vi "channel-analyzer.vi"() -> ()   [LabVIEW 2023]
uses:
  <vilib>/Utility/NIReport.llb/Report Type.ctl
  <vilib>/Platform/TimedLoop/XDataNode/timing_clust.ctl
  <vilib>/Platform/TimedLoop/XDataNode/nitl_modes.ctl
  <vilib>/Platform/TimedLoop/XDataNode/wakeup.ctl
  e44e8500-82ed-4d51-b0d7-703651abc422.vi
  <vilib>/Utility/NIReport.llb/Append Numeric Table to Report (wrap).vi
  <vilib>/Instr/_visa.llb/VISA Configure Serial Port (Instr).vi
  <vilib>/express/express analysis/Spectral/Block/exnSpectralBlock spectral measurements peak poly.vi
  <vilib>/express/express analysis/Spectral/Block/exnSpectralBlock spectral measurements peak WFM.vi
  <vilib>/platform/TimedLoop/XDataNode/XDataNode.xnode
  <vilib>/express/express analysis/Spectral/XNode/ExpressSpectralMeasurementsBlockNode.xnode
  <vilib>/Utility/NIReport.llb/NI_report.lvclass
  <vilib>/Utility/NIReport.llb/Excel/NI_Excel.lvclass
  <vilib>/Utility/NIReport.llb/NI_ReportGenerationCore.lvlib
  <vilib>/Platform/TimedLoop/XDataNode/XDNodeRunTimeDep.lvlib
panel:
  in  "Magnitude (V)":sgl min=0 max=3.3
  out "Block Size Indicator":u32
  in  "Block Size":u16(knob) min=6 max=12 scale=6.0..12.0
  in  "Start":bool
  in  "Stop Frequency (Hz)":sgl min=0 max=25000
  in  "Frequency Step (Hz)":sgl min=6.103516 max=24000
  in  "Save":bool
  in  "Start Frequency (Hz)":sgl min=1 max=25000
  out "Frequency Domain Indicator":cluster{"f0":dbl, "df":dbl, "magnitude":dbl[]}
  out "Time Domain Indicator":waveform(dbl)
  in  "Resolution (Bits)":u8 min=5 max=9
  in  "Connect":bool
  in  "Stop":bool
  in  "Reference Voltage (V)":sgl min=0
  in  "Baud Rate (BPS)":u32
  in  "COM Port":refnum<visa-resource-name>
  in  "Sampling Rate (Hz)":sgl min=0
  in  "Tab Control":enum32{"Oscilloscope", "Analyzer"}(tab)
  out "Time Domain":waveform(dbl)(graph)
  out "Frequency Domain":waveform(dbl)[](graph)
  out "Bode Plot":waveform(dbl)[](graph)
  # "CHANNEL ANALYZER"
  # "SETTINGS"
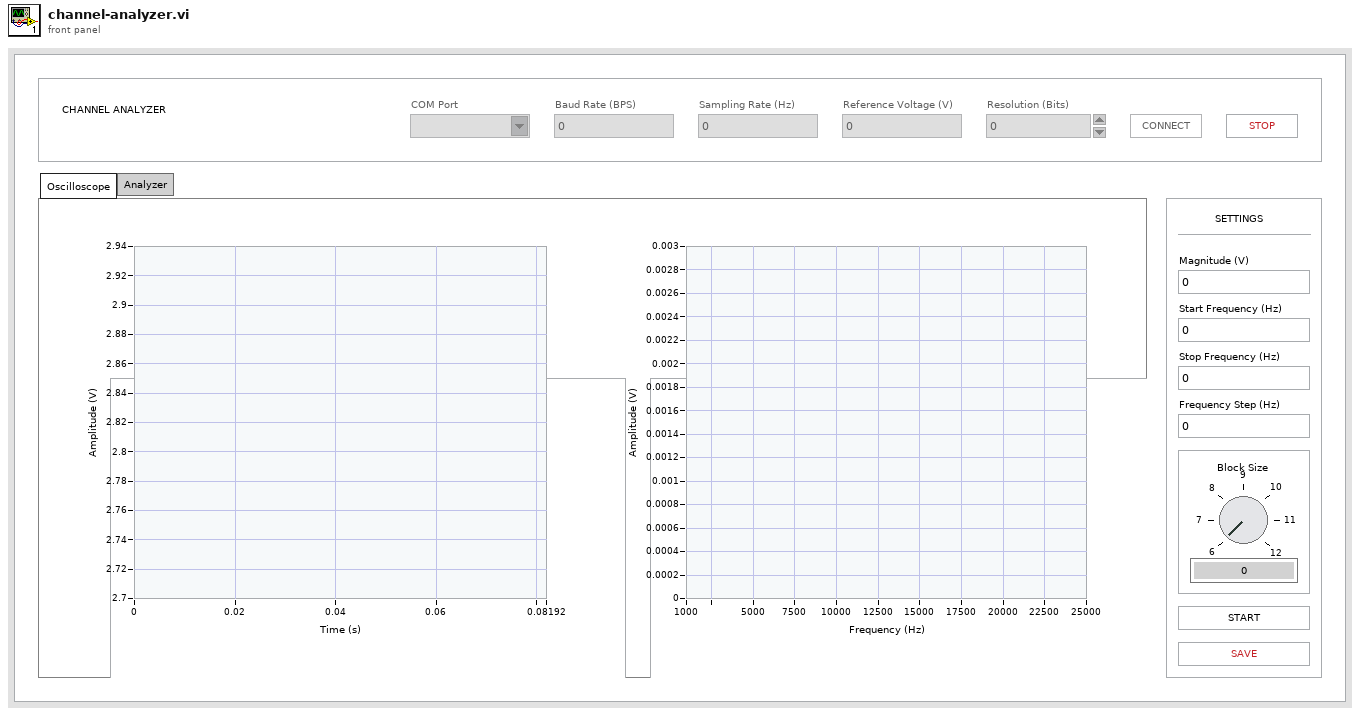
[diagram p1: front panel]
types:
  T1 = cluster{"averaging mode":u16, "weighting mode":u16, "number of averages":u32}
  T2 = cluster{"dB On (F)":bool, "unwrap phase (F)":bool, "convert to degree (F)":bool}
  T3 = enum8{"Enabled", "Disabled", "Disabled and Grayed Out"}
  T4 = typedef "NI_ReportGenerationCore.lvlib/Report Type.ctl" = enum16{"HTML", "Word", "Excel"}
  T5 = typedef "XDNodeRunTimeDep.lvlib/timing_clust.ctl" = cluster{"Expected End [f-1]":u64, "Actual End [f-1]":u64, "Finished Late? [f-1]":bool, "Expected End [i-1]":u64, "Actual End [i-1]":u64, "Finished Late? [i-1]":bool, "Expected Start [i]":u64, "Actual Start [i]":u64, "Expected Start [f]":u64, "Actual Start [f]":u64, "Source Name":string, "Structure Name":string, "Period":i64, "Deadline":i64, "Offset":i64, "Start":i64, "Priority":i32, "Timeout":i32, "Mode":T6, "Wakeup Reason":T7, "Error":errorcluster, "Source Type":string, "Secondary Source Type":string, "Global End Time":u64, "Global Start Time":u64, "Frame Duration":u64, "Iteration Duration":u64, "Assigned CPU":i32, "I/O Scan Engine Mode":u32}
  T6 = typedef "XDNodeRunTimeDep.lvlib/nitl_modes.ctl" = enum32{"No Change", "Process missed periods, maintain original phase", "Discard missed periods, maintain original phase", "Process missed periods, ignore original phase", "Discard missed periods, ignore original phase"}
  T7 = typedef "XDNodeRunTimeDep.lvlib/wakeup.ctl" = enum32{"Normal", "Aborted", "Asynchronous wakeup", "Timing source error", "Timed loop error", "Timeout"}
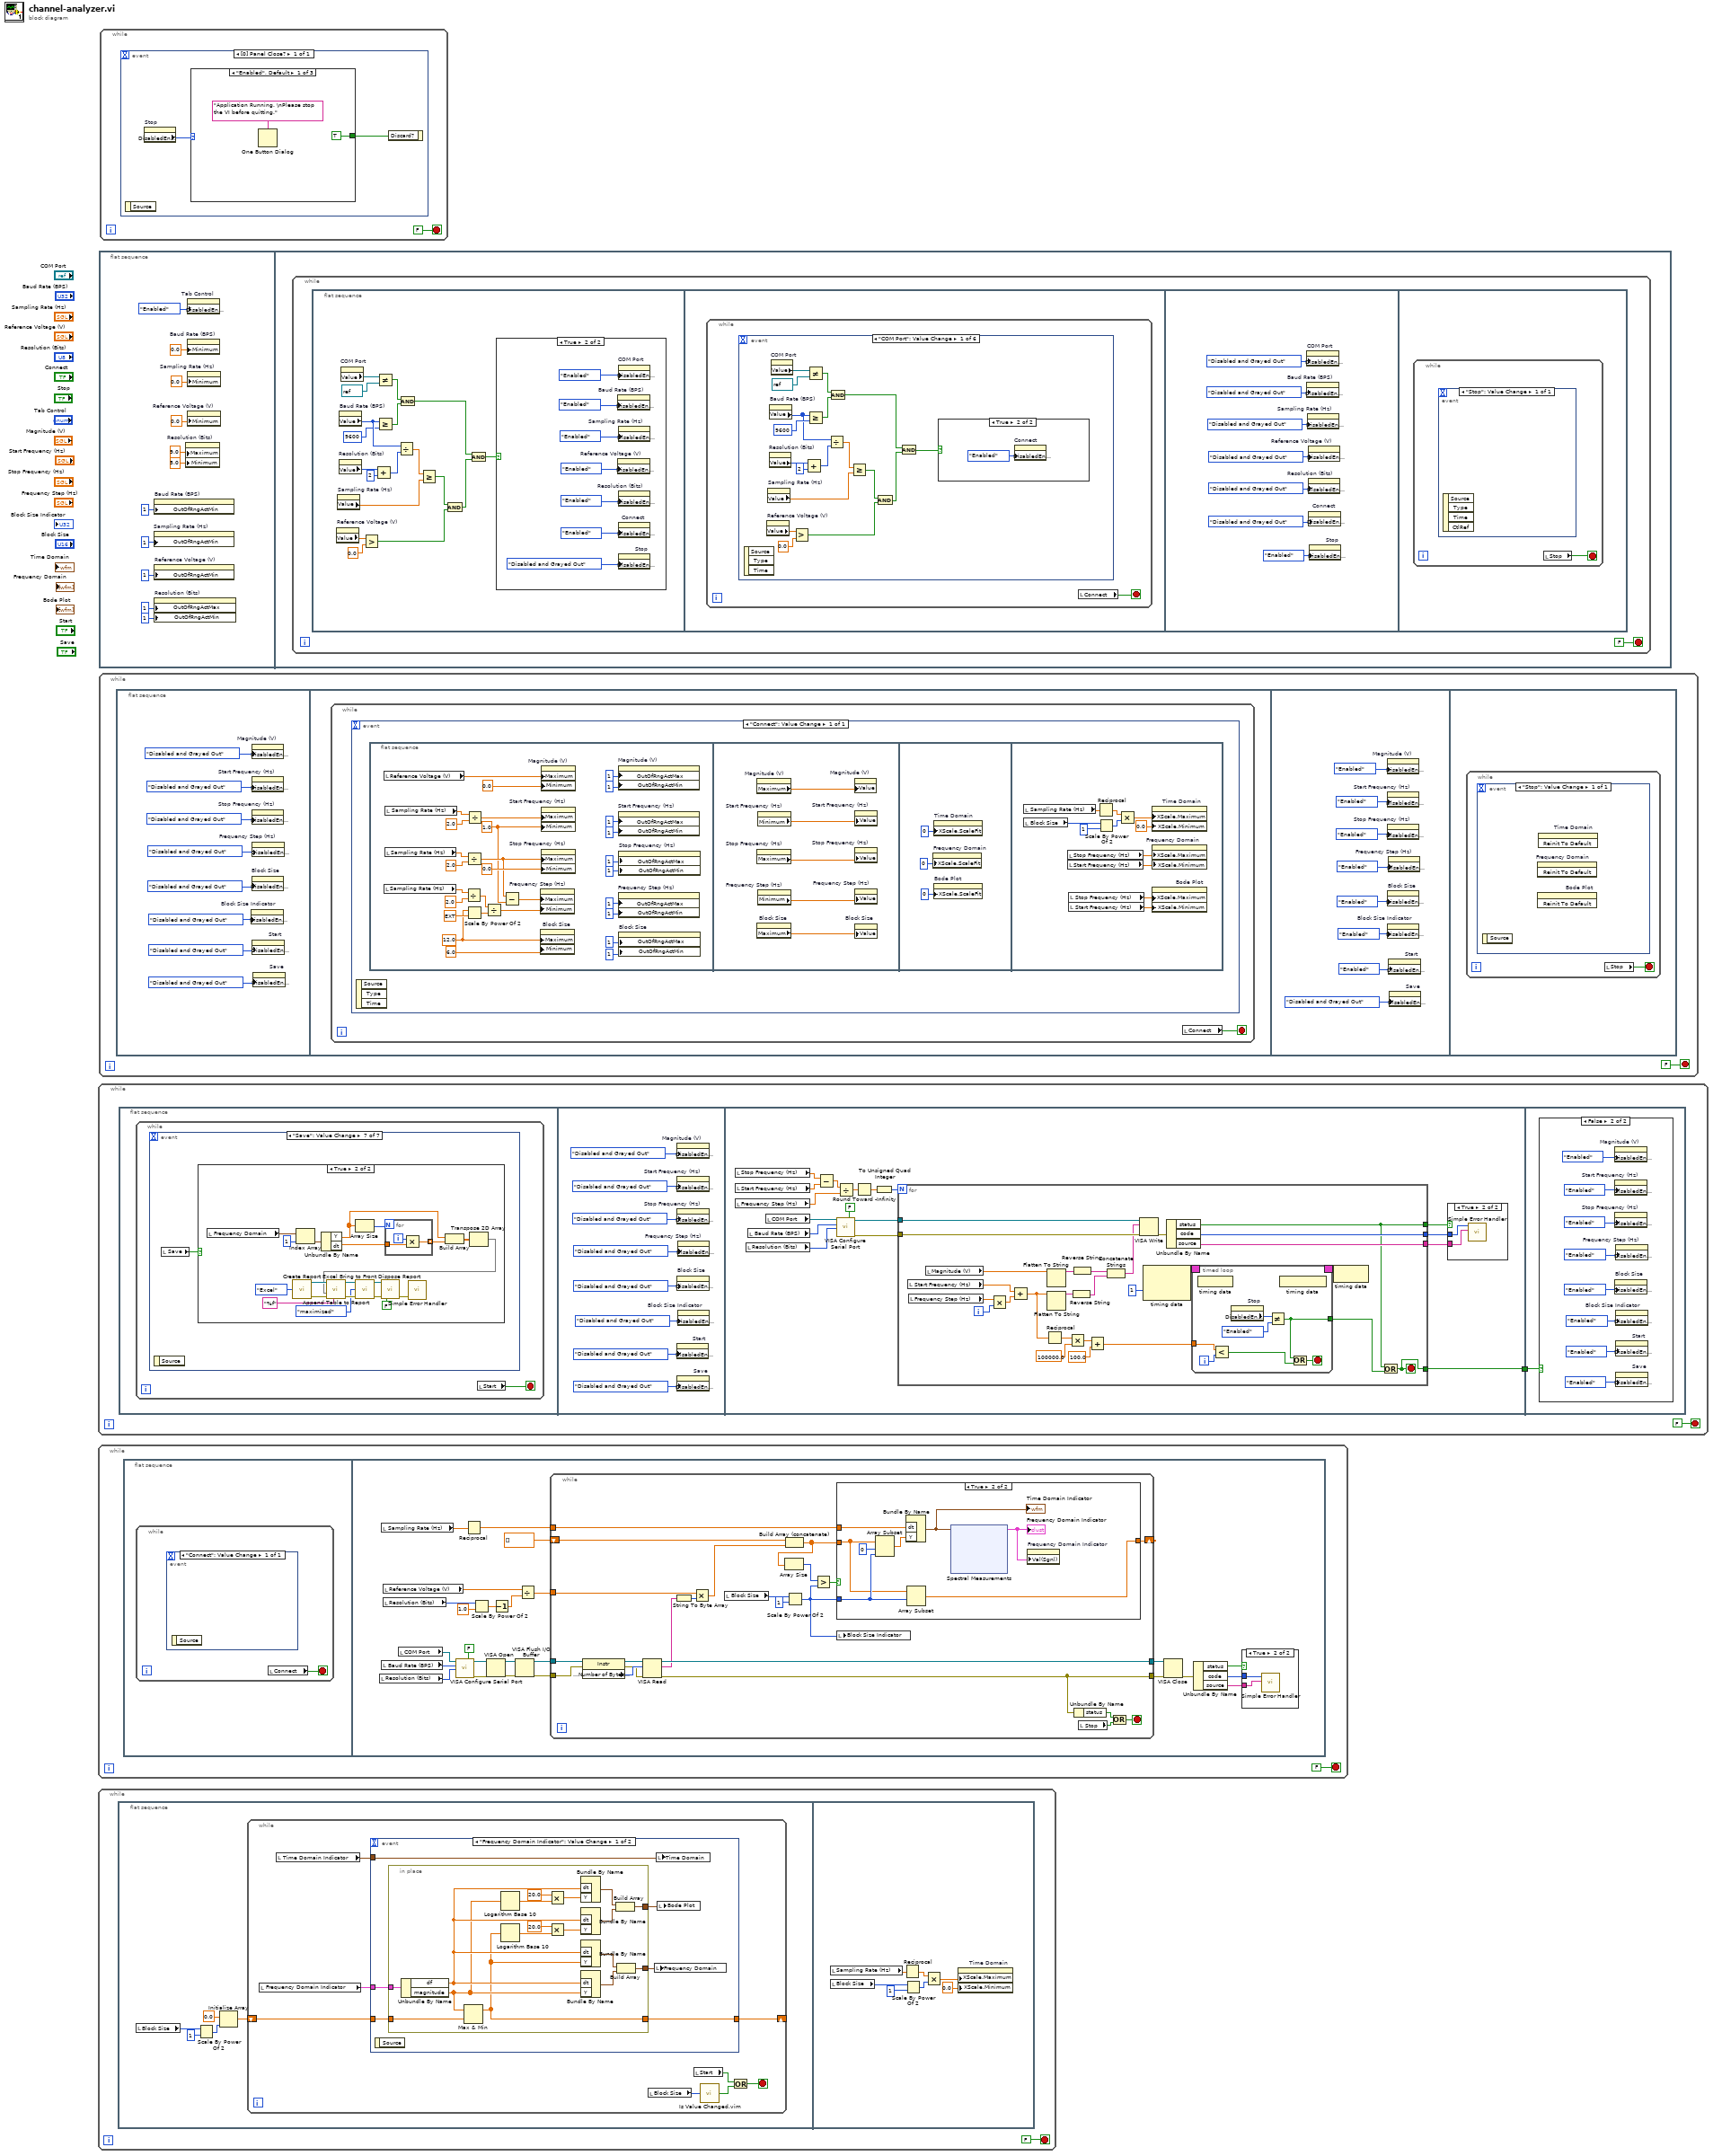
[diagram p0: block diagram]
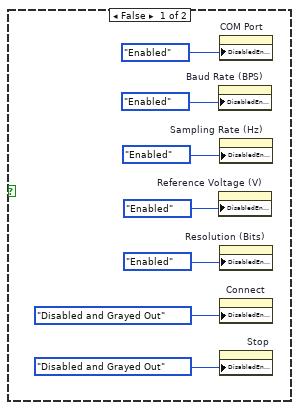
[diagram p2: hidden frame]
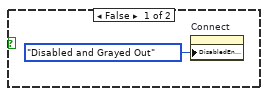
[diagram p3: hidden frame]
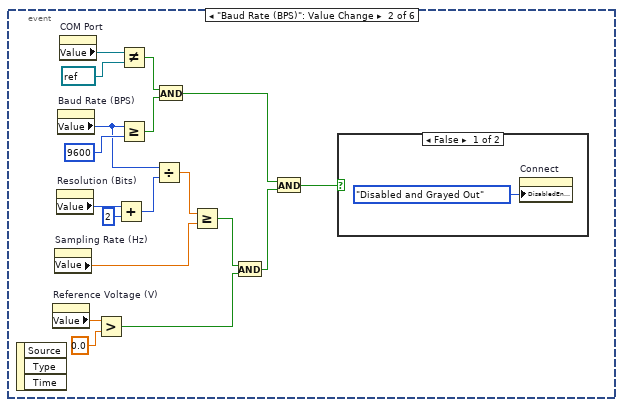
[diagram p4: hidden frame]
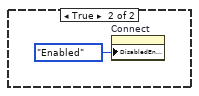
[diagram p5: hidden frame]
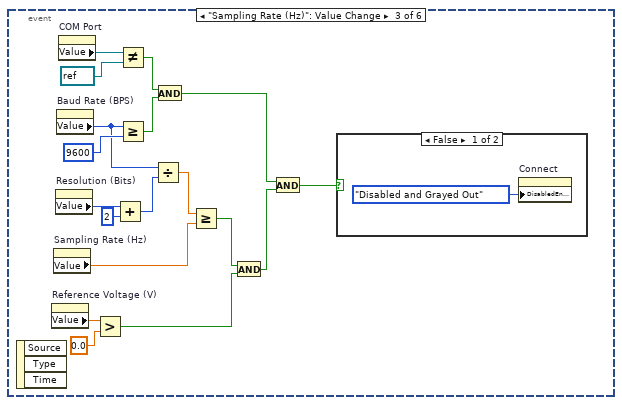
[diagram p6: hidden frame]
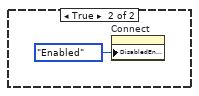
[diagram p7: hidden frame]
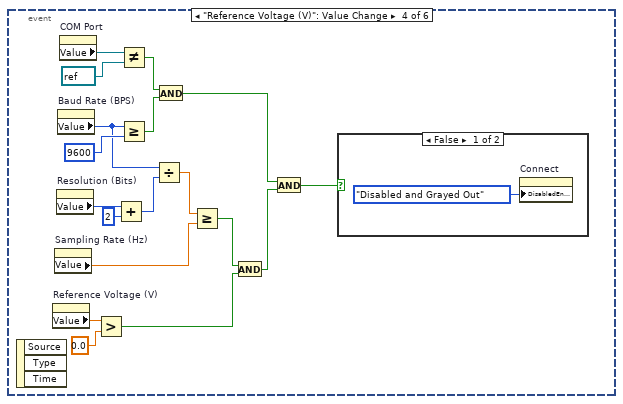
[diagram p8: hidden frame]
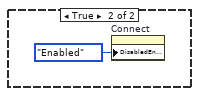
[diagram p9: hidden frame]
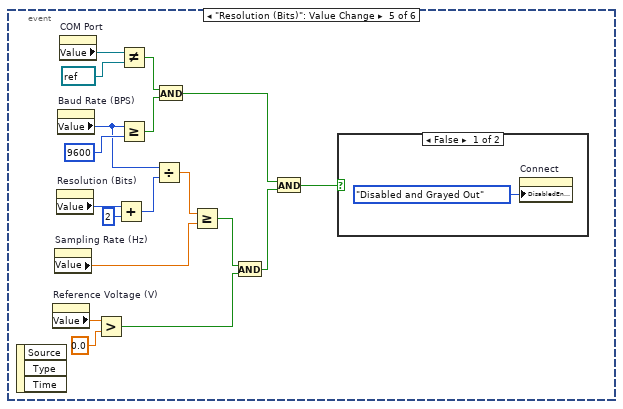
[diagram p10: hidden frame]
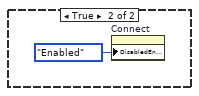
[diagram p11: hidden frame]
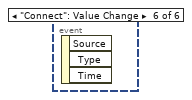
[diagram p12: hidden frame]
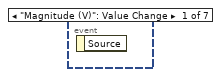
[diagram p15: hidden frame]
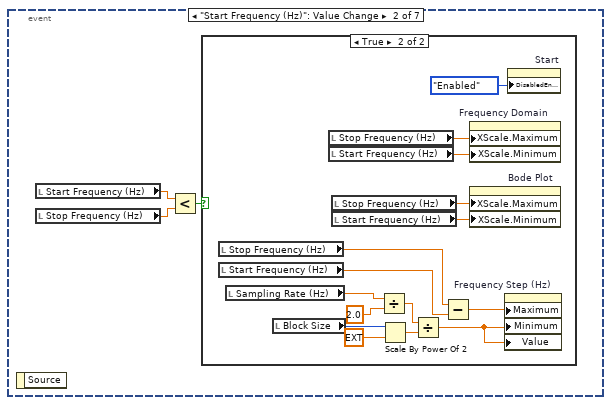
[diagram p16: hidden frame]
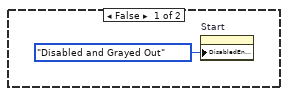
[diagram p17: hidden frame]
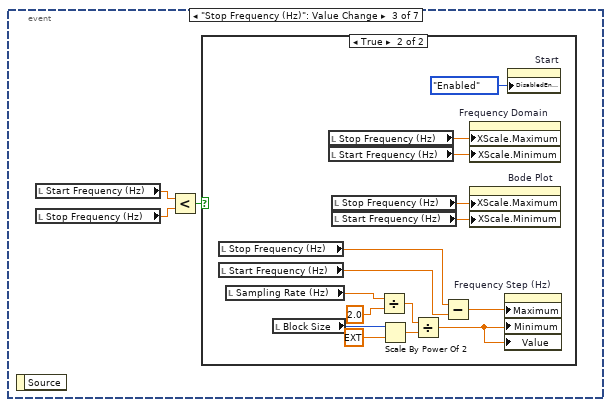
[diagram p18: hidden frame]
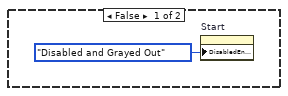
[diagram p19: hidden frame]
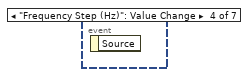
[diagram p20: hidden frame]
diagram:
  n1 = while {
    stop <- FALSE stop-if-true
    n2 = flat-sequence {
      frame #0 {
        n3 = while {
          stop <- w2 stop-if-true
          n4 = event shown="[0] \"Connect\": Value Change" {
            selector: _ -> [_]
            dyn-events: _ -> [_]
            timeout: _ -> [_]
            event "Connect": Value Change {
              n5 = event-data() -> ()  [unwired: 1 in, 1 out]
            }
          }
          n6 = local read "Connect"() -> (w2:bool)
        }
      }
      frame #1 {
        n7 = local read "Resolution (Bits)"() -> (w3:u8)
        n8 = local read "Sampling Rate (Hz)"() -> (w13:sgl)
        n9 = local read "Baud Rate (BPS)"() -> (w9:u32)
        n10 = local read "Reference Voltage (V)"() -> (w12:sgl)
        n11 = local read "Resolution (Bits)"() -> (w11:u8)
        n12 = local read "COM Port"() -> (w10:refnum<visa-resource-name>)
        n13 = call-poly "VISA Configure Serial Port"("VISA resource name"=w10, "Enable Termination\nChar (T)"=FALSE ("Enable Termination\nChar (T)"), "baud rate (9600)"=w9, "data bits (8)"=w3) -> ("VISA resource name out"=w26:refnum<visa-resource-name>, "error out"=w25:errorcluster)  [unwired: 10 in]
        n14 = Reciprocal(x=w13) -> (1/x=w22:sgl)
        n15 = Scale By Power Of 2(n=w11, x=1.0) -> (x*2^n=w16:dbl)
        n16 = VISA Open(error in (no error)=w25, VISA resource name=w26) -> (VISA resource name=w23:refnum<visa-resource-name>, error out=w24:errorcluster)  [unwired: 3 in]
        n17 = Decrement(x=w16) -> (x-1=w15:dbl)
        n18 = VISA Flush I/O Buffer(VISA resource name=w23, error in (no error)=w24) -> (VISA resource name out=w21:refnum<visa-resource-name>, error out=w20:errorcluster)  [unwired: 1 in]
        n19 = Divide(x=w12, y=w15) -> (x/y=w19:dbl)
        n20 = while {
          tunnel: w22 -> [w50]
          tunnel: w21 -> [w49]
          tunnel: w20 -> [w48]
          tunnel: w19 -> [w45]
          shift-right: [w46] -> _
          shift-left: dbl[] [] -> [w47]
          tunnel: [w44] -> w18
          tunnel: [w43] -> w8
          stop <- w29 stop-if-true
          n21 = property class="Instr"(reference=w49, error in=w48) -> (reference out=w32:refnum<visa-resource-name>, error out=w30:errorcluster, "Serial Settings:Number of Bytes at Serial Port"=w31:u32)
          n22 = VISA Read(VISA resource name=w32, byte count=w31, error in (no error)=w30) -> (VISA resource name out=w44:refnum<visa-resource-name>, read buffer=w33:string, error out=w43:errorcluster)  [unwired: 1 out]
          n23 = String To Byte Array(string=w33) -> (unsigned byte array=w38:u8[])
          n24 = Multiply(x=w45, y=w38) -> (x*y=w37:dbl[])
          n25 = local read "Block Size"() -> (w36:u16)
          n26 = Build Array (concatenate)(w47, w37) -> (w40:dbl[])
          n27 = Array Size(array=w40) -> (size(s)=w41:i32)
          n28 = Scale By Power Of 2(n=w36, x=u32 1) -> (x*2^n=w28:u32)
          n29 = Greater?(x=w41, y=w28) -> (0:w42:bool)
          n30 = case shown="True" w42 {
            tunnel: w40 -> [w51 w57]
            tunnel: [w51 w53] -> w46
            tunnel: w28 -> [_ w58]
            tunnel: w50 -> [_ w55]
            frame False {
            }
            frame True {
              n31 = Array Subset(array=w57, index=0, length=w58) -> (w56:dbl[])
              n32 = Bundle By Name("dt"=w55, "Y"=w56) -> (w54:waveform(dbl))  [unwired: 1 in]
              "Time Domain Indicator" <- w54
              n33 = Array Subset(array=w57, index=w58) -> (w53:dbl[])  [unwired: 1 in]
              n34 = xnode "Spectral Measurements"("Signals"=w54) -> ("FFT - (Peak)"=w52:cluster{"f0":dbl, "df":dbl, "magnitude":dbl[]})  [unwired: 1 in, 2 out]
              "Frequency Domain Indicator" <- w52
              n35 = property on="Frequency Domain Indicator" class="Clust (strict)"("Val(Sgnl)"=w52) -> ()  [unwired: 2 in, 2 out]
            }
          }
          n36 = local write "Block Size Indicator"(w28) -> ()
          n37 = Unbundle By Name(w43) -> ("status"=w35:bool)
          n38 = local read "Stop"() -> (w34:bool)
          n39 = Or(x=w35, y=w34) -> (x .or. y?=w29:bool)
        }
        n40 = VISA Close(VISA resource name=w18, error in (no error)=w8) -> (error out=w4:errorcluster)
        n41 = Unbundle By Name(w4) -> ("status"=w5:bool, "code"=w7:i32, "source"=w6:string)
        n42 = case shown="True" w5 {
          tunnel: w7 -> [_ w71]
          tunnel: w6 -> [_ w70]
          frame False {
          }
          frame True {
            n43 = call <vilib>:"Simple Error Handler.vi"("error code (no error:0)"=w71, "error source (\" \")"=w70) -> ()  [unwired: 3 in, 5 out]
          }
        }
      }
    }
  }
  n44 = while {
    stop <- FALSE stop-if-true
    n45 = flat-sequence {
      frame #0 {
        n46 = local read "Block Size"() -> (w75:u16)
        n47 = Scale By Power Of 2(n=w75, x=u32 1) -> (x*2^n=w73:u32)
        n48 = Initialize Array(0.0 ("element"), w73) -> (w77:dbl[])
        n49 = while {
          shift-right: [w84] -> _
          shift-left: w77 -> [w83]
          stop <- w80 stop-if-true
          n50 = local read "Frequency Domain Indicator"() -> (w85:cluster{"f0":dbl, "df":dbl, "magnitude":dbl[]})
          n51 = local read "Time Domain Indicator"() -> (w82:waveform(dbl))
          n52 = event shown="[0] \"Frequency Domain Indicator\": Value Change" {
            selector: _ -> [_ _]
            dyn-events: _ -> [_ _]
            timeout: _ -> [_ _]
            tunnel: w85 -> [w89 _]
            tunnel: w83 -> [w91 w109]
            tunnel: [w90 w109] -> w84
            tunnel: w82 -> [w88 _]
            event "Frequency Domain Indicator": Value Change {
              n53 = event-data() -> ()  [unwired: 1 in, 1 out]
              n54 = in-place {
                in-place-border: w91 -> [w108]
                in-place-border: [w92] -> w90
                in-place-border: w89 -> [w107]
                in-place-border: [w104] -> w87
                in-place-border: [w94] -> w86
                n55 = Unbundle By Name(w107) -> ("df"=w97:dbl, "magnitude"=w93:dbl[])
                n56 = Max & Min(x=w93, y=w108) -> (max(x,y)=w92:dbl[])  [unwired: 1 out]
                n57 = Logarithm Base 10(1:w93) -> (0:w101:dbl[])
                n58 = Logarithm Base 10(1:w92) -> (0:w102:dbl[])
                n59 = Multiply(x=20.0 ("y"), y=w101) -> (x*y=w99:dbl[])
                n60 = Multiply(x=20.0 ("y"), y=w102) -> (x*y=w98:dbl[])
                n61 = Bundle By Name("dt"=w97, "Y"=w99) -> (w95:waveform(dbl))  [unwired: 1 in]
                n62 = Bundle By Name("dt"=w97, "Y"=w98) -> (w96:waveform(dbl))  [unwired: 1 in]
                n63 = Bundle By Name("dt"=w97, "Y"=w92) -> (w106:waveform(dbl))  [unwired: 1 in]
                n64 = Bundle By Name("dt"=w97, "Y"=w93) -> (w105:waveform(dbl))  [unwired: 1 in]
                n65 = Build Array(w95, w96) -> (w94:waveform(dbl)[])
                n66 = Build Array(w106, w105) -> (w104:waveform(dbl)[])
              }
              n67 = local write "Frequency Domain"(w87) -> ()
              n68 = local write "Time Domain"(w88) -> ()
              n69 = local write "Bode Plot"(w86) -> ()
            }
            event "Start": Value Change {
              n70 = event-data() -> ()  [unwired: 1 in, 1 out]
            }
          }
          n71 = local read "Block Size"() -> (w81:u16)
          n72 = local read "Start"() -> (w78:bool)
          n73 = call "Is Value Changed.vim"("value"=w81) -> ("changed or first call?"=w79:bool)
          n74 = Or(x=w78, y=w79) -> (x .or. y?=w80:bool)
        }
      }
      frame #1 {
        n75 = local read "Sampling Rate (Hz)"() -> (w112:sgl)
        n76 = local read "Block Size"() -> (w114:u16)
        n77 = Reciprocal(x=w112) -> (1/x=w111:sgl)
        n78 = Scale By Power Of 2(n=w114, x=u32 1) -> (x*2^n=w116:u32)
        n79 = Multiply(x=w111, y=w116) -> (x*y=w110:sgl)
        n80 = property on="Time Domain" class="WFGraph (strict)"("XScale.Maximum"=w110, "XScale.Minimum"=0.0 ("X Scale.Range:Minimum")) -> ()  [unwired: 2 in, 2 out]
      }
    }
  }
  n81 = while {
    stop <- FALSE stop-if-true
    n82 = flat-sequence {
      tunnel: [w203] -> w117
      tunnel: w117 -> [w259]
      frame #0 {
        n83 = while {
          stop <- w119 stop-if-true
          n84 = event shown="[6] \"Save\": Value Change" {
            selector: _ -> [_ _ _ _ _ _ _]
            dyn-events: _ -> [_ _ _ _ _ _ _]
            timeout: _ -> [_ _ _ _ _ _ _]
            event "Magnitude (V)": Value Change {
              n85 = event-data() -> ()  [unwired: 1 in, 1 out]
            }
            event "Start Frequency (Hz)": Value Change {
              n86 = event-data() -> ()  [unwired: 1 in, 1 out]
              n87 = local read "Start Frequency (Hz)"() -> (w121:sgl)
              n88 = local read "Stop Frequency (Hz)"() -> (w120:sgl)
              n89 = Less?(x=w121, y=w120) -> (x < y?=w122:bool)
              n90 = case shown="True" w122 {
                frame False {
                  n91 = property on="Start" class="Bool (strict)"("DisabledEnum"=T3."Disabled and Grayed Out" ("Disabled")) -> ()  [unwired: 2 in, 2 out]
                }
                frame True {
                  n92 = local read "Stop Frequency (Hz)"() -> (w128:sgl)
                  n93 = local read "Start Frequency (Hz)"() -> (w127:sgl)
                  n94 = local read "Sampling Rate (Hz)"() -> (w131:sgl)
                  n95 = local read "Block Size"() -> (w129:u16)
                  n96 = local read "Stop Frequency (Hz)"() -> (w135:sgl)
                  n97 = local read "Start Frequency (Hz)"() -> (w134:sgl)
                  n98 = local read "Stop Frequency (Hz)"() -> (w136:sgl)
                  n99 = local read "Start Frequency (Hz)"() -> (w137:sgl)
                  n100 = Divide(x=w131, y=sgl 2.0) -> (x/y=w132:sgl)
                  n101 = Scale By Power Of 2(n=w129, x=ext 1.0) -> (x*2^n=w130:ext)
                  n102 = Divide(x=w132, y=w130) -> (x/y=w126:ext)
                  n103 = Subtract(x=w128, y=w127) -> (x-y=w133:sgl)
                  n104 = property on="Frequency Domain" class="WFGraph (strict)"("XScale.Maximum"=w135, "XScale.Minimum"=w134) -> ()  [unwired: 2 in, 2 out]
                  n105 = property on="Bode Plot" class="WFGraph (strict)"("XScale.Maximum"=w136, "XScale.Minimum"=w137) -> ()  [unwired: 2 in, 2 out]
                  n106 = property on="Frequency Step (Hz)" class="DigNum (strict)"("Maximum"=w133, "Minimum"=w126, "Value"=w126) -> ()  [unwired: 2 in, 2 out]
                  n107 = property on="Start" class="Bool (strict)"("DisabledEnum"=T3."Enabled" ("Disabled")) -> ()  [unwired: 2 in, 2 out]
                }
              }
            }
            event "Stop Frequency (Hz)": Value Change {
              n108 = event-data() -> ()  [unwired: 1 in, 1 out]
              n109 = local read "Start Frequency (Hz)"() -> (w140:sgl)
              n110 = local read "Stop Frequency (Hz)"() -> (w139:sgl)
              n111 = Less?(x=w140, y=w139) -> (x < y?=w141:bool)
              n112 = case shown="True" w141 {
                frame False {
                  n113 = property on="Start" class="Bool (strict)"("DisabledEnum"=T3."Disabled and Grayed Out" ("Disabled")) -> ()  [unwired: 2 in, 2 out]
                }
                frame True {
                  n114 = local read "Stop Frequency (Hz)"() -> (w147:sgl)
                  n115 = local read "Start Frequency (Hz)"() -> (w146:sgl)
                  n116 = local read "Sampling Rate (Hz)"() -> (w150:sgl)
                  n117 = local read "Block Size"() -> (w148:u16)
                  n118 = local read "Stop Frequency (Hz)"() -> (w154:sgl)
                  n119 = local read "Start Frequency (Hz)"() -> (w153:sgl)
                  n120 = local read "Stop Frequency (Hz)"() -> (w155:sgl)
                  n121 = local read "Start Frequency (Hz)"() -> (w156:sgl)
                  n122 = Divide(x=w150, y=sgl 2.0) -> (x/y=w151:sgl)
                  n123 = Scale By Power Of 2(n=w148, x=ext 1.0) -> (x*2^n=w149:ext)
                  n124 = Divide(x=w151, y=w149) -> (x/y=w145:ext)
                  n125 = Subtract(x=w147, y=w146) -> (x-y=w152:sgl)
                  n126 = property on="Frequency Domain" class="WFGraph (strict)"("XScale.Maximum"=w154, "XScale.Minimum"=w153) -> ()  [unwired: 2 in, 2 out]
                  n127 = property on="Bode Plot" class="WFGraph (strict)"("XScale.Maximum"=w155, "XScale.Minimum"=w156) -> ()  [unwired: 2 in, 2 out]
                  n128 = property on="Frequency Step (Hz)" class="DigNum (strict)"("Maximum"=w152, "Minimum"=w145, "Value"=w145) -> ()  [unwired: 2 in, 2 out]
                  n129 = property on="Start" class="Bool (strict)"("DisabledEnum"=T3."Enabled" ("Disabled")) -> ()  [unwired: 2 in, 2 out]
                }
              }
            }
            event "Frequency Step (Hz)": Value Change {
              n130 = event-data() -> ()  [unwired: 1 in, 1 out]
            }
            event "Block Size": Value Change {
              n131 = event-data() -> ()  [unwired: 1 in, 1 out]
              n132 = local read "Stop Frequency (Hz)"() -> (w160:sgl)
              n133 = local read "Start Frequency (Hz)"() -> (w159:sgl)
              n134 = local read "Sampling Rate (Hz)"() -> (w165:sgl)
              n135 = local read "Block Size"() -> (w162:u16)
              n136 = Divide(x=w165, y=sgl 2.0) -> (x/y=w166:sgl)
              n137 = Scale By Power Of 2(n=w162, x=ext 1.0) -> (x*2^n=w163:ext)
              n138 = Divide(x=w166, y=w163) -> (x/y=w158:ext)
              n139 = Subtract(x=w160, y=w159) -> (x-y=w167:sgl)
              n140 = property on="Frequency Step (Hz)" class="DigNum (strict)"("Maximum"=w167, "Minimum"=w158, "Value"=w158) -> ()  [unwired: 2 in, 2 out]
            }
            event "Start": Value Change {
              n141 = event-data() -> ()  [unwired: 1 in, 1 out]
            }
            event "Save": Value Change {
              n142 = event-data() -> ()  [unwired: 1 in, 1 out]
              n143 = local read "Save"() -> (w168:bool)
              n144 = case shown="True" w168 {
                frame False {
                }
                frame True {
                  n145 = local read "Frequency Domain"() -> (w181:waveform(dbl)[])
                  n146 = call <vilib>:"Create Report.vi"("report type"=Report_Type."Excel") -> ("report out"=w185:refnum<class "NI_report.lvclass">, "error out"=w184:errorcluster)  [unwired: 13 in]
                  n147 = Index Array(array=w181, index=1) -> (element=w179:waveform(dbl))
                  n148 = Unbundle By Name(w179) -> ("Y"=w169:dbl[], "dt"=w177:dbl)
                  n149 = Array Size(array=w169) -> (size(s)=w171:i32)
                  n150 = for {
                    N: w171 -> [_]
                    tunnel: w177 -> [w190]
                    tunnel: [w189] -> w176 mode=indexing
                    i -> [w191]
                    n151 = Multiply(x=w191, y=w190) -> (x*y=w189:dbl)
                  }
                  n152 = Build Array(w169, w176) -> (w174:dbl[][])
                  n153 = Transpose 2D Array(2D array=w174) -> (transposed array=w173:dbl[][])
                  n154 = call-poly <vilib>:"Append Table to Report.vi"("report in"=w185, "numerical data"=w173, "error in (no error)"=w184, "format string (%.3f)"="%f") -> ("report out"=w183:refnum<class "NI_report.lvclass">, "error out"=w182:errorcluster)  [unwired: 8 in, 2 out]
                  n155 = call <vilib>:"Excel Bring to Front.vi"("report in"=w183, "window state (maximized)"=enum16{"maximized", "minimized", "normal"}."maximized", "error in (no error)"=w182) -> ("report out"=w188:refnum<class "NI_report.lvclass">, "error out"=w187:errorcluster)  [unwired: 11 in]
                  n156 = call-dynamic "Dispose Report.vi"("report in"=w188, "error in (no error)"=w187, "close report? (T)"=FALSE) -> ("error out"=w178:errorcluster)  [unwired: 12 in]
                  n157 = call <vilib>:"Simple Error Handler.vi"("error in (no error)"=w178) -> ()  [unwired: 4 in, 5 out]
                }
              }
            }
          }
          n158 = local read "Start"() -> (w119:bool)
        }
      }
      frame #1 {
        n159 = property on="Start" class="Bool (strict)"("DisabledEnum"=T3."Disabled and Grayed Out" ("Disabled")) -> ()  [unwired: 2 in, 2 out]
        n160 = property on="Magnitude (V)" class="DigNum (strict)"("DisabledEnum"=T3."Disabled and Grayed Out" ("Disabled")) -> ()  [unwired: 2 in, 2 out]
        n161 = property on="Start Frequency (Hz)" class="DigNum (strict)"("DisabledEnum"=T3."Disabled and Grayed Out" ("Disabled")) -> ()  [unwired: 2 in, 2 out]
        n162 = property on="Stop Frequency (Hz)" class="DigNum (strict)"("DisabledEnum"=T3."Disabled and Grayed Out" ("Disabled")) -> ()  [unwired: 2 in, 2 out]
        n163 = property on="Block Size" class="Knob (strict)"("DisabledEnum"=T3."Disabled and Grayed Out" ("Disabled")) -> ()  [unwired: 2 in, 2 out]
        n164 = property on="Save" class="Bool (strict)"("DisabledEnum"=T3."Disabled and Grayed Out" ("Disabled")) -> ()  [unwired: 2 in, 2 out]
        n165 = property on="Frequency Step (Hz)" class="DigNum (strict)"("DisabledEnum"=T3."Disabled and Grayed Out" ("Disabled")) -> ()  [unwired: 2 in, 2 out]
        n166 = property on="Block Size Indicator" class="DigNum (strict)"("DisabledEnum"=T3."Disabled and Grayed Out" ("Disabled")) -> ()  [unwired: 2 in, 2 out]
      }
      frame #2 {
        n167 = local read "Stop Frequency (Hz)"() -> (w208:sgl)
        n168 = local read "Start Frequency (Hz)"() -> (w207:sgl)
        n169 = local read "Frequency Step (Hz)"() -> (w212:sgl)
        n170 = local read "Resolution (Bits)"() -> (w204:u8)
        n171 = local read "Baud Rate (BPS)"() -> (w216:u32)
        n172 = local read "COM Port"() -> (w215:refnum<visa-resource-name>)
        n173 = Subtract(x=w208, y=w207) -> (x-y=w213:sgl)
        n174 = call-poly "VISA Configure Serial Port"("VISA resource name"=w215, "Enable Termination\nChar (T)"=FALSE ("Enable Termination\nChar (T)"), "baud rate (9600)"=w216, "data bits (8)"=w204) -> ("VISA resource name out"=w210:refnum<visa-resource-name>, "error out"=w209:errorcluster)  [unwired: 10 in]
        n175 = Divide(x=w213, y=w212) -> (x/y=w211:sgl)
        n176 = Round Toward -Infinity(1:w211) -> (0:w206:sgl)
        n177 = To Unsigned Quad Integer(1:w206) -> (0:w205:u64)
        n178 = for {
          N: w205 -> [_]
          tunnel: w210 -> [w245]
          tunnel: w209 -> [w244]
          tunnel: [w231] -> w203
          tunnel: [w232] -> w202
          tunnel: [w241] -> w201
          tunnel: [w240] -> w200
          i -> [w227]
          stop <- w231 stop-if-true
          n179 = local read "Start Frequency (Hz)"() -> (w236:sgl)
          n180 = local read "Frequency Step (Hz)"() -> (w238:sgl)
          n181 = local read "Magnitude (V)"() -> (w239:sgl)
          n182 = Multiply(x=w238, y=w227) -> (x*y=w237:sgl)
          n183 = Add(x=w236, y=w237) -> (x+y=w235:sgl)
          n184 = Reciprocal(x=w235) -> (1/x=w222:sgl)
          n185 = Flatten To String(anything=w239) -> (data string=w226:string)  [unwired: 3 in, 2 out]
          n186 = Flatten To String(anything=w235) -> (data string=w225:string)  [unwired: 3 in, 2 out]
          n187 = Multiply(x=w222, y=sgl 100000.0) -> (x*y=w220:sgl)
          n188 = Reverse String(1:w225) -> (0:w224:string)
          n189 = Reverse String(1:w226) -> (0:w223:string)
          n190 = Add(x=w220, y=sgl 100.0) -> (x+y=w229:sgl)
          n191 = Concatenate Strings(w223, w224) -> (w243:string)
          n192 = VISA Write(VISA resource name=w245, write buffer=w243, error in (no error)=w244) -> (error out=w242:errorcluster)  [unwired: 2 out]
          n193 = node-c288(i64 1 ("Period")) -> (w234:T5)  [unwired: 1 in]
          n194 = Unbundle By Name(w242) -> ("status"=w232:bool, "code"=w241:i32, "source"=w240:string)
          n195 = timed-loop {
            timing: w234 -> [_]
            timing-out: [_] -> w233
            tunnel: [w249] -> w230
            tunnel: w229 -> [w248]
            i -> [w247]
            stop <- w250 stop-if-true
            n196 = node-c288() -> ()  [unwired: 1 in]
            n197 = Less?(x=w248, y=w247) -> (x < y?=w246:bool)
            n198 = property on="Stop" class="Bool (strict)"() -> ("DisabledEnum"=w252:T3)  [unwired: 2 in, 2 out]
            n199 = Not Equal?(x=w252, y=T3."Enabled" ("Disabled")) -> (x != y?=w249:bool)
            n200 = node-c288() -> ()  [unwired: 1 out]
            n201 = Or(x=w249, y=w246) -> (x .or. y?=w250:bool)
          }
          n202 = node-c288(w233) -> ()
          n203 = Or(x=w232, y=w230) -> (x .or. y?=w231:bool)
        }
        n204 = case shown="True" w202 {
          tunnel: w201 -> [_ w218]
          tunnel: w200 -> [_ w217]
          frame False {
          }
          frame True {
            n205 = call <vilib>:"Simple Error Handler.vi"("error code (no error:0)"=w218, "error source (\" \")"=w217) -> ()  [unwired: 3 in, 5 out]
          }
        }
      }
      frame #3 {
        n206 = case shown="False" w259 {
          frame True {
          }
          frame False {
            n207 = property on="Magnitude (V)" class="DigNum (strict)"("DisabledEnum"=T3."Enabled" ("Disabled")) -> ()  [unwired: 2 in, 2 out]
            n208 = property on="Start Frequency (Hz)" class="DigNum (strict)"("DisabledEnum"=T3."Enabled" ("Disabled")) -> ()  [unwired: 2 in, 2 out]
            n209 = property on="Stop Frequency (Hz)" class="DigNum (strict)"("DisabledEnum"=T3."Enabled" ("Disabled")) -> ()  [unwired: 2 in, 2 out]
            n210 = property on="Block Size" class="Knob (strict)"("DisabledEnum"=T3."Enabled" ("Disabled")) -> ()  [unwired: 2 in, 2 out]
            n211 = property on="Frequency Step (Hz)" class="DigNum (strict)"("DisabledEnum"=T3."Enabled" ("Disabled")) -> ()  [unwired: 2 in, 2 out]
            n212 = property on="Block Size Indicator" class="DigNum (strict)"("DisabledEnum"=T3."Enabled" ("Disabled")) -> ()  [unwired: 2 in, 2 out]
            n213 = property on="Start" class="Bool (strict)"("DisabledEnum"=T3."Enabled" ("Disabled")) -> ()  [unwired: 2 in, 2 out]
            n214 = property on="Save" class="Bool (strict)"("DisabledEnum"=T3."Enabled" ("Disabled")) -> ()  [unwired: 2 in, 2 out]
          }
        }
      }
    }
  }
  n215 = flat-sequence {
    frame #0 {
      n216 = property on="Sampling Rate (Hz)" class="DigNum (strict)"("OutOfRngActMin"=u8 1 ("Response to Value Outside Limits:Minimum")) -> ()  [unwired: 2 in, 2 out]
      n217 = property on="Baud Rate (BPS)" class="DigNum (strict)"("OutOfRngActMin"=u8 1 ("Response to Value Outside Limits:Minimum")) -> ()  [unwired: 2 in, 2 out]
      n218 = property on="Reference Voltage (V)" class="DigNum (strict)"("OutOfRngActMin"=u8 1 ("Response to Value Outside Limits:Minimum")) -> ()  [unwired: 2 in, 2 out]
      n219 = property on="Resolution (Bits)" class="DigNum (strict)"("OutOfRngActMax"=u8 1 ("Response to Value Outside Limits:Maximum"), "OutOfRngActMin"=u8 1 ("Response to Value Outside Limits:Minimum")) -> ()  [unwired: 2 in, 2 out]
      n220 = property on="Resolution (Bits)" class="DigNum (strict)"("Maximum"=9.0 ("Data Entry Limits:Maximum"), "Minimum"=5.0 ("Data Entry Limits:Minimum")) -> ()  [unwired: 2 in, 2 out]
      n221 = property on="Baud Rate (BPS)" class="DigNum (strict)"("Minimum"=0.0 ("Data Entry Limits:Minimum")) -> ()  [unwired: 2 in, 2 out]
      n222 = property on="Tab Control" class="TabCtl (strict)"("DisabledEnum"=T3."Enabled" ("Disabled")) -> ()  [unwired: 2 in, 2 out]
      n223 = property on="Sampling Rate (Hz)" class="DigNum (strict)"("Minimum"=0.0 ("Data Entry Limits:Minimum")) -> ()  [unwired: 2 in, 2 out]
      n224 = property on="Reference Voltage (V)" class="DigNum (strict)"("Minimum"=0.0 ("Data Entry Limits:Minimum")) -> ()  [unwired: 2 in, 2 out]
    }
    frame #1 {
      n225 = while {
        stop <- FALSE stop-if-true
        n226 = flat-sequence {
          frame #0 {
            n227 = property on="Reference Voltage (V)" class="DigNum (strict)"() -> ("Value"=w284:sgl)  [unwired: 2 in, 2 out]
            n228 = property on="Sampling Rate (Hz)" class="DigNum (strict)"() -> ("Value"=w291:sgl)  [unwired: 2 in, 2 out]
            n229 = property on="Resolution (Bits)" class="DigNum (strict)"() -> ("Value"=w286:u8)  [unwired: 2 in, 2 out]
            n230 = property on="Baud Rate (BPS)" class="DigNum (strict)"() -> ("Value"=w289:u32)  [unwired: 2 in, 2 out]
            n231 = property on="COM Port" class="VISAName"() -> ("Value"=w282:refnum<visa-resource-name>)  [unwired: 2 in, 2 out]
            n232 = Greater?(x=w284, y=sgl 0.0) -> (0:w293:bool)
            n233 = Add(x=w286, y=u8 2) -> (x+y=w288:u8)
            n234 = Not Equal?(x=w282, y=refnum<visa-resource-name> refnum ("COM Port")) -> (x != y?=w295:bool)
            n235 = Greater Or Equal?(x=w289, y=u32 9600) -> (x >= y?=w294:bool)
            n236 = Divide(x=w289, y=w288) -> (x/y=w290:dbl)
            n237 = And(x=w295, y=w294) -> (x .and. y?=w296:bool)
            n238 = Greater Or Equal?(x=w290, y=w291) -> (x >= y?=w292:bool)
            n239 = And(x=w292, y=w293) -> (x .and. y?=w297:bool)
            n240 = And(x=w296, y=w297) -> (x .and. y?=w281:bool)
            n241 = case shown="True" w281 {
              frame False {
                n242 = property on="Baud Rate (BPS)" class="DigNum (strict)"("DisabledEnum"=T3."Enabled" ("Disabled")) -> ()  [unwired: 2 in, 2 out]
                n243 = property on="Reference Voltage (V)" class="DigNum (strict)"("DisabledEnum"=T3."Enabled" ("Disabled")) -> ()  [unwired: 2 in, 2 out]
                n244 = property on="COM Port" class="VISAName"("DisabledEnum"=T3."Enabled" ("Disabled")) -> ()  [unwired: 2 in, 2 out]
                n245 = property on="Sampling Rate (Hz)" class="DigNum (strict)"("DisabledEnum"=T3."Enabled" ("Disabled")) -> ()  [unwired: 2 in, 2 out]
                n246 = property on="Resolution (Bits)" class="DigNum (strict)"("DisabledEnum"=T3."Enabled" ("Disabled")) -> ()  [unwired: 2 in, 2 out]
                n247 = property on="Connect" class="Bool (strict)"("DisabledEnum"=T3."Disabled and Grayed Out" ("Disabled")) -> ()  [unwired: 2 in, 2 out]
                n248 = property on="Stop" class="Bool (strict)"("DisabledEnum"=T3."Disabled and Grayed Out" ("Disabled")) -> ()  [unwired: 2 in, 2 out]
              }
              frame True {
                n249 = property on="Baud Rate (BPS)" class="DigNum (strict)"("DisabledEnum"=T3."Enabled" ("Disabled")) -> ()  [unwired: 2 in, 2 out]
                n250 = property on="Reference Voltage (V)" class="DigNum (strict)"("DisabledEnum"=T3."Enabled" ("Disabled")) -> ()  [unwired: 2 in, 2 out]
                n251 = property on="COM Port" class="VISAName"("DisabledEnum"=T3."Enabled" ("Disabled")) -> ()  [unwired: 2 in, 2 out]
                n252 = property on="Sampling Rate (Hz)" class="DigNum (strict)"("DisabledEnum"=T3."Enabled" ("Disabled")) -> ()  [unwired: 2 in, 2 out]
                n253 = property on="Resolution (Bits)" class="DigNum (strict)"("DisabledEnum"=T3."Enabled" ("Disabled")) -> ()  [unwired: 2 in, 2 out]
                n254 = property on="Connect" class="Bool (strict)"("DisabledEnum"=T3."Enabled" ("Disabled")) -> ()  [unwired: 2 in, 2 out]
                n255 = property on="Stop" class="Bool (strict)"("DisabledEnum"=T3."Disabled and Grayed Out" ("Disabled")) -> ()  [unwired: 2 in, 2 out]
              }
            }
          }
          frame #1 {
            n256 = while {
              stop <- w312 stop-if-true
              n257 = event shown="[0] \"COM Port\": Value Change" {
                selector: _ -> [_ _ _ _ _ _]
                dyn-events: _ -> [_ _ _ _ _ _]
                timeout: _ -> [_ _ _ _ _ _]
                event "COM Port": Value Change {
                  n258 = event-data() -> ()  [unwired: 1 in, 3 out]
                  n259 = property on="Reference Voltage (V)" class="DigNum (strict)"() -> ("Value"=w328:sgl)  [unwired: 2 in, 2 out]
                  n260 = property on="Sampling Rate (Hz)" class="DigNum (strict)"() -> ("Value"=w320:sgl)  [unwired: 2 in, 2 out]
                  n261 = property on="Resolution (Bits)" class="DigNum (strict)"() -> ("Value"=w325:u8)  [unwired: 2 in, 2 out]
                  n262 = property on="Baud Rate (BPS)" class="DigNum (strict)"() -> ("Value"=w322:u32)  [unwired: 2 in, 2 out]
                  n263 = property on="COM Port" class="VISAName"() -> ("Value"=w330:refnum<visa-resource-name>)  [unwired: 2 in, 2 out]
                  n264 = Greater?(x=w328, y=sgl 0.0) -> (0:w318:bool)
                  n265 = Add(x=w325, y=u8 2) -> (x+y=w323:u8)
                  n266 = Not Equal?(x=w330, y=refnum<visa-resource-name> refnum ("COM Port")) -> (x != y?=w316:bool)
                  n267 = Greater Or Equal?(x=w322, y=u32 9600) -> (x >= y?=w317:bool)
                  n268 = Divide(x=w322, y=w323) -> (x/y=w321:dbl)
                  n269 = And(x=w316, y=w317) -> (x .and. y?=w315:bool)
                  n270 = Greater Or Equal?(x=w321, y=w320) -> (x >= y?=w319:bool)
                  n271 = And(x=w319, y=w318) -> (x .and. y?=w314:bool)
                  n272 = And(x=w315, y=w314) -> (x .and. y?=w313:bool)
                  n273 = case shown="True" w313 {
                    frame False {
                      n274 = property on="Connect" class="Bool (strict)"("DisabledEnum"=T3."Disabled and Grayed Out" ("Disabled")) -> ()  [unwired: 2 in, 2 out]
                    }
                    frame True {
                      n275 = property on="Connect" class="Bool (strict)"("DisabledEnum"=T3."Enabled" ("Disabled")) -> ()  [unwired: 2 in, 2 out]
                    }
                  }
                }
                event "Baud Rate (BPS)": Value Change {
                  n276 = event-data() -> ()  [unwired: 1 in, 3 out]
                  n277 = property on="Reference Voltage (V)" class="DigNum (strict)"() -> ("Value"=w348:sgl)  [unwired: 2 in, 2 out]
                  n278 = property on="Sampling Rate (Hz)" class="DigNum (strict)"() -> ("Value"=w340:sgl)  [unwired: 2 in, 2 out]
                  n279 = property on="Resolution (Bits)" class="DigNum (strict)"() -> ("Value"=w345:u8)  [unwired: 2 in, 2 out]
                  n280 = property on="Baud Rate (BPS)" class="DigNum (strict)"() -> ("Value"=w342:u32)  [unwired: 2 in, 2 out]
                  n281 = property on="COM Port" class="VISAName"() -> ("Value"=w350:refnum<visa-resource-name>)  [unwired: 2 in, 2 out]
                  n282 = Greater?(x=w348, y=sgl 0.0) -> (0:w338:bool)
                  n283 = Add(x=w345, y=u8 2) -> (x+y=w343:u8)
                  n284 = Not Equal?(x=w350, y=refnum<visa-resource-name> refnum ("COM Port")) -> (x != y?=w336:bool)
                  n285 = Greater Or Equal?(x=w342, y=u32 9600) -> (x >= y?=w337:bool)
                  n286 = Divide(x=w342, y=w343) -> (x/y=w341:dbl)
                  n287 = And(x=w336, y=w337) -> (x .and. y?=w335:bool)
                  n288 = Greater Or Equal?(x=w341, y=w340) -> (x >= y?=w339:bool)
                  n289 = And(x=w339, y=w338) -> (x .and. y?=w334:bool)
                  n290 = And(x=w335, y=w334) -> (x .and. y?=w333:bool)
                  n291 = case shown="False" w333 {
                    frame False {
                      n292 = property on="Connect" class="Bool (strict)"("DisabledEnum"=T3."Disabled and Grayed Out" ("Disabled")) -> ()  [unwired: 2 in, 2 out]
                    }
                    frame True {
                      n293 = property on="Connect" class="Bool (strict)"("DisabledEnum"=T3."Enabled" ("Disabled")) -> ()  [unwired: 2 in, 2 out]
                    }
                  }
                }
                event "Sampling Rate (Hz)": Value Change {
                  n294 = event-data() -> ()  [unwired: 1 in, 3 out]
                  n295 = property on="Reference Voltage (V)" class="DigNum (strict)"() -> ("Value"=w368:sgl)  [unwired: 2 in, 2 out]
                  n296 = property on="Sampling Rate (Hz)" class="DigNum (strict)"() -> ("Value"=w360:sgl)  [unwired: 2 in, 2 out]
                  n297 = property on="Resolution (Bits)" class="DigNum (strict)"() -> ("Value"=w365:u8)  [unwired: 2 in, 2 out]
                  n298 = property on="Baud Rate (BPS)" class="DigNum (strict)"() -> ("Value"=w362:u32)  [unwired: 2 in, 2 out]
                  n299 = property on="COM Port" class="VISAName"() -> ("Value"=w370:refnum<visa-resource-name>)  [unwired: 2 in, 2 out]
                  n300 = Greater?(x=w368, y=sgl 0.0) -> (0:w358:bool)
                  n301 = Add(x=w365, y=u8 2) -> (x+y=w363:u8)
                  n302 = Not Equal?(x=w370, y=refnum<visa-resource-name> refnum ("COM Port")) -> (x != y?=w356:bool)
                  n303 = Greater Or Equal?(x=w362, y=u32 9600) -> (x >= y?=w357:bool)
                  n304 = Divide(x=w362, y=w363) -> (x/y=w361:dbl)
                  n305 = And(x=w356, y=w357) -> (x .and. y?=w355:bool)
                  n306 = Greater Or Equal?(x=w361, y=w360) -> (x >= y?=w359:bool)
                  n307 = And(x=w359, y=w358) -> (x .and. y?=w354:bool)
                  n308 = And(x=w355, y=w354) -> (x .and. y?=w353:bool)
                  n309 = case shown="False" w353 {
                    frame False {
                      n310 = property on="Connect" class="Bool (strict)"("DisabledEnum"=T3."Disabled and Grayed Out" ("Disabled")) -> ()  [unwired: 2 in, 2 out]
                    }
                    frame True {
                      n311 = property on="Connect" class="Bool (strict)"("DisabledEnum"=T3."Enabled" ("Disabled")) -> ()  [unwired: 2 in, 2 out]
                    }
                  }
                }
                event "Reference Voltage (V)": Value Change {
                  n312 = event-data() -> ()  [unwired: 1 in, 3 out]
                  n313 = property on="Reference Voltage (V)" class="DigNum (strict)"() -> ("Value"=w388:sgl)  [unwired: 2 in, 2 out]
                  n314 = property on="Sampling Rate (Hz)" class="DigNum (strict)"() -> ("Value"=w380:sgl)  [unwired: 2 in, 2 out]
                  n315 = property on="Resolution (Bits)" class="DigNum (strict)"() -> ("Value"=w385:u8)  [unwired: 2 in, 2 out]
                  n316 = property on="Baud Rate (BPS)" class="DigNum (strict)"() -> ("Value"=w382:u32)  [unwired: 2 in, 2 out]
                  n317 = property on="COM Port" class="VISAName"() -> ("Value"=w390:refnum<visa-resource-name>)  [unwired: 2 in, 2 out]
                  n318 = Greater?(x=w388, y=sgl 0.0) -> (0:w378:bool)
                  n319 = Add(x=w385, y=u8 2) -> (x+y=w383:u8)
                  n320 = Not Equal?(x=w390, y=refnum<visa-resource-name> refnum ("COM Port")) -> (x != y?=w376:bool)
                  n321 = Greater Or Equal?(x=w382, y=u32 9600) -> (x >= y?=w377:bool)
                  n322 = Divide(x=w382, y=w383) -> (x/y=w381:dbl)
                  n323 = And(x=w376, y=w377) -> (x .and. y?=w375:bool)
                  n324 = Greater Or Equal?(x=w381, y=w380) -> (x >= y?=w379:bool)
                  n325 = And(x=w379, y=w378) -> (x .and. y?=w374:bool)
                  n326 = And(x=w375, y=w374) -> (x .and. y?=w373:bool)
                  n327 = case shown="False" w373 {
                    frame False {
                      n328 = property on="Connect" class="Bool (strict)"("DisabledEnum"=T3."Disabled and Grayed Out" ("Disabled")) -> ()  [unwired: 2 in, 2 out]
                    }
                    frame True {
                      n329 = property on="Connect" class="Bool (strict)"("DisabledEnum"=T3."Enabled" ("Disabled")) -> ()  [unwired: 2 in, 2 out]
                    }
                  }
                }
                event "Resolution (Bits)": Value Change {
                  n330 = event-data() -> ()  [unwired: 1 in, 3 out]
                  n331 = property on="Reference Voltage (V)" class="DigNum (strict)"() -> ("Value"=w408:sgl)  [unwired: 2 in, 2 out]
                  n332 = property on="Sampling Rate (Hz)" class="DigNum (strict)"() -> ("Value"=w400:sgl)  [unwired: 2 in, 2 out]
                  n333 = property on="Resolution (Bits)" class="DigNum (strict)"() -> ("Value"=w405:u8)  [unwired: 2 in, 2 out]
                  n334 = property on="Baud Rate (BPS)" class="DigNum (strict)"() -> ("Value"=w402:u32)  [unwired: 2 in, 2 out]
                  n335 = property on="COM Port" class="VISAName"() -> ("Value"=w410:refnum<visa-resource-name>)  [unwired: 2 in, 2 out]
                  n336 = Greater?(x=w408, y=sgl 0.0) -> (0:w398:bool)
                  n337 = Add(x=w405, y=u8 2) -> (x+y=w403:u8)
                  n338 = Not Equal?(x=w410, y=refnum<visa-resource-name> refnum ("COM Port")) -> (x != y?=w396:bool)
                  n339 = Greater Or Equal?(x=w402, y=u32 9600) -> (x >= y?=w397:bool)
                  n340 = Divide(x=w402, y=w403) -> (x/y=w401:dbl)
                  n341 = And(x=w396, y=w397) -> (x .and. y?=w395:bool)
                  n342 = Greater Or Equal?(x=w401, y=w400) -> (x >= y?=w399:bool)
                  n343 = And(x=w399, y=w398) -> (x .and. y?=w394:bool)
                  n344 = And(x=w395, y=w394) -> (x .and. y?=w393:bool)
                  n345 = case shown="False" w393 {
                    frame False {
                      n346 = property on="Connect" class="Bool (strict)"("DisabledEnum"=T3."Disabled and Grayed Out" ("Disabled")) -> ()  [unwired: 2 in, 2 out]
                    }
                    frame True {
                      n347 = property on="Connect" class="Bool (strict)"("DisabledEnum"=T3."Enabled" ("Disabled")) -> ()  [unwired: 2 in, 2 out]
                    }
                  }
                }
                event "Connect": Value Change {
                  n348 = event-data() -> ()  [unwired: 1 in, 3 out]
                }
              }
              n349 = local read "Connect"() -> (w312:bool)
            }
          }
          frame #2 {
            n350 = property on="COM Port" class="VISAName"("DisabledEnum"=T3."Disabled and Grayed Out" ("Disabled")) -> ()  [unwired: 2 in, 2 out]
            n351 = property on="Baud Rate (BPS)" class="DigNum (strict)"("DisabledEnum"=T3."Disabled and Grayed Out" ("Disabled")) -> ()  [unwired: 2 in, 2 out]
            n352 = property on="Sampling Rate (Hz)" class="DigNum (strict)"("DisabledEnum"=T3."Disabled and Grayed Out" ("Disabled")) -> ()  [unwired: 2 in, 2 out]
            n353 = property on="Reference Voltage (V)" class="DigNum (strict)"("DisabledEnum"=T3."Disabled and Grayed Out" ("Disabled")) -> ()  [unwired: 2 in, 2 out]
            n354 = property on="Resolution (Bits)" class="DigNum (strict)"("DisabledEnum"=T3."Disabled and Grayed Out" ("Disabled")) -> ()  [unwired: 2 in, 2 out]
            n355 = property on="Connect" class="Bool (strict)"("DisabledEnum"=T3."Disabled and Grayed Out" ("Disabled")) -> ()  [unwired: 2 in, 2 out]
            n356 = property on="Stop" class="Bool (strict)"("DisabledEnum"=T3."Enabled" ("Disabled")) -> ()  [unwired: 2 in, 2 out]
          }
          frame #3 {
            n357 = while {
              stop <- w420 stop-if-true
              n358 = event shown="[0] \"Stop\": Value Change" {
                selector: _ -> [_]
                dyn-events: _ -> [_]
                timeout: _ -> [_]
                event "Stop": Value Change {
                  n359 = event-data() -> ()  [unwired: 1 in, 4 out]
                }
              }
              n360 = local read "Stop"() -> (w420:bool)
            }
          }
        }
      }
    }
  }
  n361 = while {
    stop <- FALSE stop-if-true
    n362 = flat-sequence {
      frame #0 {
        n363 = property on="Block Size Indicator" class="DigNum (strict)"("DisabledEnum"=T3."Disabled and Grayed Out" ("Disabled")) -> ()  [unwired: 2 in, 2 out]
        n364 = property on="Magnitude (V)" class="DigNum (strict)"("DisabledEnum"=T3."Disabled and Grayed Out" ("Disabled")) -> ()  [unwired: 2 in, 2 out]
        n365 = property on="Start Frequency (Hz)" class="DigNum (strict)"("DisabledEnum"=T3."Disabled and Grayed Out" ("Disabled")) -> ()  [unwired: 2 in, 2 out]
        n366 = property on="Stop Frequency (Hz)" class="DigNum (strict)"("DisabledEnum"=T3."Disabled and Grayed Out" ("Disabled")) -> ()  [unwired: 2 in, 2 out]
        n367 = property on="Block Size" class="Knob (strict)"("DisabledEnum"=T3."Disabled and Grayed Out" ("Disabled")) -> ()  [unwired: 2 in, 2 out]
        n368 = property on="Frequency Step (Hz)" class="DigNum (strict)"("DisabledEnum"=T3."Disabled and Grayed Out" ("Disabled")) -> ()  [unwired: 2 in, 2 out]
        n369 = property on="Start" class="Bool (strict)"("DisabledEnum"=T3."Disabled and Grayed Out" ("Disabled")) -> ()  [unwired: 2 in, 2 out]
        n370 = property on="Save" class="Bool (strict)"("DisabledEnum"=T3."Disabled and Grayed Out" ("Disabled")) -> ()  [unwired: 2 in, 2 out]
      }
      frame #1 {
        n371 = while {
          stop <- w430 stop-if-true
          n372 = event shown="[0] \"Connect\": Value Change" {
            selector: _ -> [_]
            dyn-events: _ -> [_]
            timeout: _ -> [_]
            event "Connect": Value Change {
              n373 = event-data() -> ()  [unwired: 1 in, 3 out]
              n374 = flat-sequence {
                frame #0 {
                  w431 = 12.0 ("Data Entry Limits:Maximum")
                  w432 = 1.0 ("Data Entry Limits:Minimum")
                  n375 = local read "Reference Voltage (V)"() -> (w455:sgl)
                  n376 = local read "Sampling Rate (Hz)"() -> (w449:sgl)
                  n377 = local read "Sampling Rate (Hz)"() -> (w458:sgl)
                  n378 = local read "Sampling Rate (Hz)"() -> (w459:sgl)
                  n379 = Divide(x=w449, y=sgl 2.0) -> (x/y=w448:sgl)
                  n380 = Divide(x=w458, y=sgl 2.0) -> (x/y=w444:sgl)
                  n381 = Scale By Power Of 2(n=w431, x=ext 1.0) -> (x*2^n=w451:ext)
                  n382 = Divide(x=w459, y=sgl 2.0) -> (x/y=w445:sgl)
                  n383 = Divide(x=w448, y=w451) -> (x/y=w447:ext)
                  n384 = Subtract(x=w444, y=w432) -> (x-y=w446:dbl)
                  n385 = property on="Frequency Step (Hz)" class="DigNum (strict)"("Maximum"=w446, "Minimum"=w447) -> ()  [unwired: 2 in, 2 out]
                  n386 = property on="Block Size" class="Knob (strict)"("Maximum"=w431, "Minimum"=6.0 ("Data Entry Limits:Minimum")) -> ()  [unwired: 2 in, 2 out]
                  n387 = property on="Magnitude (V)" class="DigNum (strict)"("Maximum"=w455, "Minimum"=0.0 ("Data Entry Limits:Minimum")) -> ()  [unwired: 2 in, 2 out]
                  n388 = property on="Start Frequency (Hz)" class="DigNum (strict)"("Maximum"=w445, "Minimum"=w432) -> ()  [unwired: 2 in, 2 out]
                  n389 = property on="Stop Frequency (Hz)" class="DigNum (strict)"("Maximum"=w444, "Minimum"=0.0 ("Data Entry Limits:Minimum")) -> ()  [unwired: 2 in, 2 out]
                  n390 = property on="Magnitude (V)" class="DigNum (strict)"("OutOfRngActMax"=u8 1 ("Response to Value Outside Limits:Maximum"), "OutOfRngActMin"=u8 1 ("Response to Value Outside Limits:Minimum")) -> ()  [unwired: 2 in, 2 out]
                  n391 = property on="Start Frequency (Hz)" class="DigNum (strict)"("OutOfRngActMax"=u8 1 ("Response to Value Outside Limits:Maximum"), "OutOfRngActMin"=u8 1 ("Response to Value Outside Limits:Minimum")) -> ()  [unwired: 2 in, 2 out]
                  n392 = property on="Frequency Step (Hz)" class="DigNum (strict)"("OutOfRngActMax"=u8 1 ("Response to Value Outside Limits:Maximum"), "OutOfRngActMin"=u8 1 ("Response to Value Outside Limits:Minimum")) -> ()  [unwired: 2 in, 2 out]
                  n393 = property on="Stop Frequency (Hz)" class="DigNum (strict)"("OutOfRngActMax"=u8 1 ("Response to Value Outside Limits:Maximum"), "OutOfRngActMin"=u8 1 ("Response to Value Outside Limits:Minimum")) -> ()  [unwired: 2 in, 2 out]
                  n394 = property on="Block Size" class="Knob (strict)"("OutOfRngActMax"=u8 1 ("Response to Value Outside Limits:Maximum"), "OutOfRngActMin"=u8 1 ("Response to Value Outside Limits:Minimum")) -> ()  [unwired: 2 in, 2 out]
                }
                frame #1 {
                  n395 = property on="Magnitude (V)" class="DigNum (strict)"() -> ("Maximum"=w463:dbl)  [unwired: 2 in, 2 out]
                  n396 = property on="Stop Frequency (Hz)" class="DigNum (strict)"() -> ("Maximum"=w461:dbl)  [unwired: 2 in, 2 out]
                  n397 = property on="Block Size" class="Knob (strict)"() -> ("Maximum"=w464:dbl)  [unwired: 2 in, 2 out]
                  n398 = property on="Start Frequency (Hz)" class="DigNum (strict)"() -> ("Minimum"=w462:dbl)  [unwired: 2 in, 2 out]
                  n399 = property on="Frequency Step (Hz)" class="DigNum (strict)"() -> ("Minimum"=w460:dbl)  [unwired: 2 in, 2 out]
                  n400 = property on="Magnitude (V)" class="DigNum (strict)"("Value"=w463) -> ()  [unwired: 2 in, 2 out]
                  n401 = property on="Start Frequency (Hz)" class="DigNum (strict)"("Value"=w462) -> ()  [unwired: 2 in, 2 out]
                  n402 = property on="Stop Frequency (Hz)" class="DigNum (strict)"("Value"=w461) -> ()  [unwired: 2 in, 2 out]
                  n403 = property on="Frequency Step (Hz)" class="DigNum (strict)"("Value"=w460) -> ()  [unwired: 2 in, 2 out]
                  n404 = property on="Block Size" class="Knob (strict)"("Value"=w464) -> ()  [unwired: 2 in, 2 out]
                }
                frame #2 {
                  n405 = property on="Frequency Domain" class="WFGraph (strict)"("XScale.ScaleFit"=u8 0 ("X Scale.Scale Fit")) -> ()  [unwired: 2 in, 2 out]
                  n406 = property on="Time Domain" class="WFGraph (strict)"("XScale.ScaleFit"=u8 0 ("X Scale.Scale Fit")) -> ()  [unwired: 2 in, 2 out]
                  n407 = property on="Bode Plot" class="WFGraph (strict)"("XScale.ScaleFit"=u8 0 ("X Scale.Scale Fit")) -> ()  [unwired: 2 in, 2 out]
                }
                frame #3 {
                  n408 = local read "Sampling Rate (Hz)"() -> (w476:sgl)
                  n409 = local read "Block Size"() -> (w470:u16)
                  n410 = local read "Stop Frequency (Hz)"() -> (w474:sgl)
                  n411 = local read "Start Frequency (Hz)"() -> (w475:sgl)
                  n412 = local read "Stop Frequency (Hz)"() -> (w472:sgl)
                  n413 = local read "Start Frequency (Hz)"() -> (w471:sgl)
                  n414 = Reciprocal(x=w476) -> (1/x=w477:sgl)
                  n415 = Scale By Power Of 2(n=w470, x=u32 1) -> (x*2^n=w468:u32)
                  n416 = Multiply(x=w477, y=w468) -> (x*y=w478:sgl)
                  n417 = property on="Time Domain" class="WFGraph (strict)"("XScale.Maximum"=w478, "XScale.Minimum"=0.0 ("X Scale.Range:Minimum")) -> ()  [unwired: 2 in, 2 out]
                  n418 = property on="Bode Plot" class="WFGraph (strict)"("XScale.Maximum"=w472, "XScale.Minimum"=w471) -> ()  [unwired: 2 in, 2 out]
                  n419 = property on="Frequency Domain" class="WFGraph (strict)"("XScale.Maximum"=w474, "XScale.Minimum"=w475) -> ()  [unwired: 2 in, 2 out]
                }
              }
            }
          }
          n420 = local read "Connect"() -> (w430:bool)
        }
      }
      frame #2 {
        n421 = property on="Magnitude (V)" class="DigNum (strict)"("DisabledEnum"=T3."Enabled" ("Disabled")) -> ()  [unwired: 2 in, 2 out]
        n422 = property on="Start Frequency (Hz)" class="DigNum (strict)"("DisabledEnum"=T3."Enabled" ("Disabled")) -> ()  [unwired: 2 in, 2 out]
        n423 = property on="Stop Frequency (Hz)" class="DigNum (strict)"("DisabledEnum"=T3."Enabled" ("Disabled")) -> ()  [unwired: 2 in, 2 out]
        n424 = property on="Block Size" class="Knob (strict)"("DisabledEnum"=T3."Enabled" ("Disabled")) -> ()  [unwired: 2 in, 2 out]
        n425 = property on="Block Size Indicator" class="DigNum (strict)"("DisabledEnum"=T3."Enabled" ("Disabled")) -> ()  [unwired: 2 in, 2 out]
        n426 = property on="Frequency Step (Hz)" class="DigNum (strict)"("DisabledEnum"=T3."Enabled" ("Disabled")) -> ()  [unwired: 2 in, 2 out]
        n427 = property on="Start" class="Bool (strict)"("DisabledEnum"=T3."Enabled" ("Disabled")) -> ()  [unwired: 2 in, 2 out]
        n428 = property on="Save" class="Bool (strict)"("DisabledEnum"=T3."Disabled and Grayed Out" ("Disabled")) -> ()  [unwired: 2 in, 2 out]
      }
      frame #3 {
        n429 = while {
          stop <- w487 stop-if-true
          n430 = event shown="[0] \"Stop\": Value Change" {
            selector: _ -> [_]
            dyn-events: _ -> [_]
            timeout: _ -> [_]
            event "Stop": Value Change {
              n431 = event-data() -> ()  [unwired: 1 in, 1 out]
              n432 = invoke on="Frequency Domain" class="WFGraph (strict)" method="Reinit To Default"() -> ()  [unwired: 3 in, 3 out]
              n433 = invoke on="Bode Plot" class="WFGraph (strict)" method="Reinit To Default"() -> ()  [unwired: 3 in, 3 out]
              n434 = invoke on="Time Domain" class="WFGraph (strict)" method="Reinit To Default"() -> ()  [unwired: 3 in, 3 out]
            }
          }
          n435 = local read "Stop"() -> (w487:bool)
        }
      }
    }
  }
  n436 = while {
    stop <- FALSE stop-if-true
    n437 = event shown="[0] Panel Close?" {
      selector: _ -> [_]
      dyn-events: _ -> [_]
      timeout: _ -> [_]
      event Panel Close? {
        n438 = event-data() -> ()  [unwired: 1 in, 1 out]
        n439 = property on="Stop" class="Bool (strict)"() -> ("DisabledEnum"=w490:T3)  [unwired: 2 in, 2 out]
        n440 = case shown="\"Enabled\", Default" w490 {
          tunnel: [TRUE ("Discard?") FALSE ("Discard?") FALSE ("Discard?")] -> w489
          frame "Enabled", Default {
            n441 = One Button Dialog(message="Application Running. \nPlease stop the VI before quitting.") -> ()  [unwired: 1 in, 1 out]
          }
          frame "Disabled" {
            n442 = Quit LabVIEW(quit? (T)=TRUE) -> ()
          }
          frame "Disabled and Grayed Out" {
            n443 = Quit LabVIEW(quit? (T)=TRUE) -> ()
          }
        }
        n444 = event-data("Discard?"=w489) -> ()  [unwired: 1 in, 1 out]
      }
    }
  }
